vi "c_Open.vi"() -> (1 "Case Label":T1="Open")   [LabVIEW 2020, in "Server Client.lvclass"]
uses:
  Server Client.lvclass
  <vilib>/addons/_Workers/Library/Case Label.ctl
  <vilib>/addons/_Workers/Library/Workers.lvlib
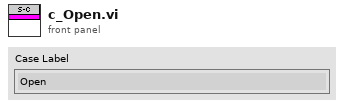
[diagram p1: front panel]
types:
  T1 = typedef "Workers.lvlib/Case Label.ctl" = string
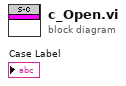
[diagram p0: block diagram]
diagram:
